vi "Root and Extension.vi"(1 "File name in":path) -> (0 "File name out":path)   [LabVIEW 2018]
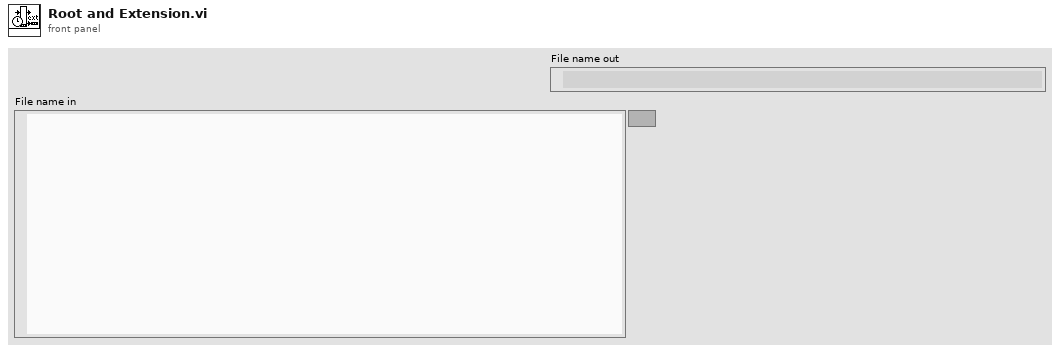
[diagram p1: front panel]
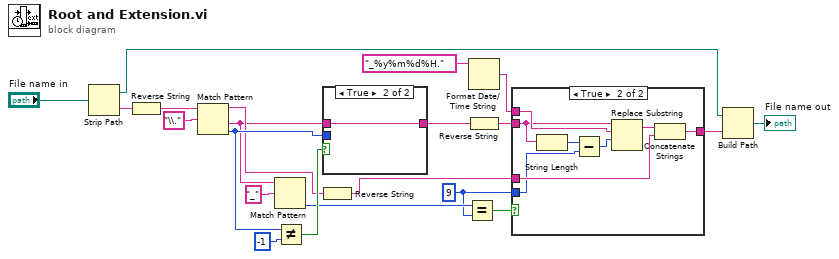
[diagram p0: block diagram]
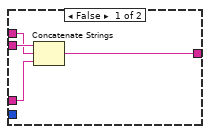
[diagram p2: hidden frame]
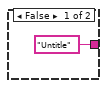
[diagram p3: hidden frame]
diagram:
  w1 = 9 ("y")
  n1 = Strip Path(path="File name in") -> (stripped path=w9:path, name=w11:string)
  n2 = Reverse String(1:w11) -> (0:w21:string)
  n3 = Match Pattern(string=w21, regular expression="\\.") -> (before substring=w12:string, after substring=w4:string, offset past match=w19:i32)  [unwired: 1 in, 1 out]
  n4 = Match Pattern(string=w4, regular expression="_") -> (offset past match=w3:i32)  [unwired: 1 in, 3 out]
  n5 = Not Equal?(x=w19, y=-1) -> (x != y?=w18:bool)
  n6 = Reverse String(1:w12) -> (0:w6:string)
  n7 = case "Has Period?" shown="True" w18 {
    tunnel: ["Untitle" w23] -> w20
    tunnel: w19 -> [_ _]
    tunnel: w4 -> [_ w23]
    frame False {
    }
    frame True {
    }
  }
  n8 = Equal?(x=w3, y=w1) -> (x = y?=w2:bool)
  n9 = Format Date/Time String(time format string (%c)="_%y%m%d%H.") -> (date/time string=w13:string)  [unwired: 2 in]
  n10 = Reverse String(1:w20) -> (0:w15:string)
  n11 = case shown="True" w2 {
    tunnel: w15 -> [w27 w31]
    tunnel: w13 -> [w26 w33]
    tunnel: [w25 w34] -> w10
    tunnel: w6 -> [w24 w35]
    tunnel: w1 -> [_ w29]
    frame False {
      n12 = Concatenate Strings(w27, w26, w24) -> (w25:string)
    }
    frame True {
      n13 = String Length(string=w31) -> (length=w30:i32)
      n14 = Subtract(x=w30, y=w29) -> (x-y=w28:i32)
      n15 = Replace Substring(3:w28, 4:w33, 5:w31) -> (1:w32:string)  [unwired: 1 in, 1 out]
      n16 = Concatenate Strings(w32, w35) -> (w34:string)
    }
  }
  n17 = Build Path(base path=w9, name or relative path=w10) -> (appended path=→"File name out":path)
